vi "Variant Array Decimate.vi"(8 "error in (no error)":errorcluster, 11 "N Dim Array":variant) -> (0 "error out":errorcluster, 1 "Variant Array Type":variant, 2 "Element Type":variant, 3 "Array of Variant Arrays":variant[](array[variant]))   [LabVIEW 2018, in "labview_json.lvlib"]
uses:
  labview_json.lvlib
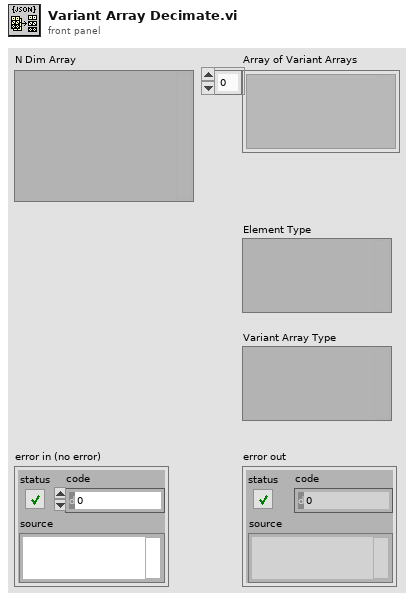
[diagram p1: front panel]
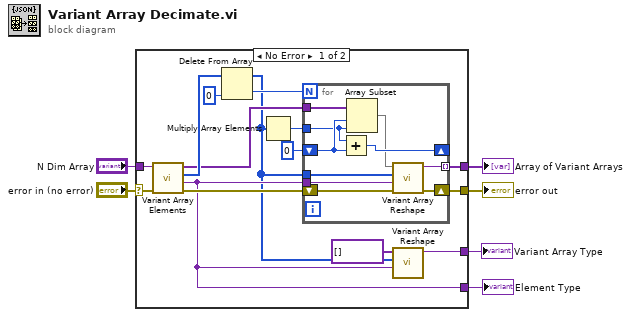
[diagram p0: block diagram]
diagram:
  n1 = case shown="No Error" "error in (no error)" {
    selector: "error in (no error)" -> [w20 w32]
    tunnel: "N Dim Array" -> [w21 _]
    tunnel: [w14 w32] -> w4
    tunnel: [w13 _] -> w3
    tunnel: [w10 _] -> w2
    tunnel: [w7 _] -> w1
    frame No Error {
      n2 = call "Variant Array Elements.vi"("error in (no error)"=w20, "N Dim Array"=w21) -> ("error out"=w12:errorcluster, "Element Type"=w10:variant, "Sizes"=w19:i32[], "Elements"=w11:variant[])  [unwired: 6 in]
      n3 = Delete From Array(array=w19, index=0) -> (deleted portion=w15:i32, array with subset deleted=w9:i32[])  [unwired: 1 in]
      n4 = Multiply Array Elements(1:w9) -> (0:w16:i32)
      n5 = for {
        N: w15 -> [_]
        tunnel: w11 -> [w31]
        shift-right: [w28] -> _
        shift-left: 0 -> [w30]
        tunnel: w16 -> [w29]
        tunnel: w9 -> [w25]
        shift-right: [w26] -> w14
        shift-left: w12 -> [w27]
        tunnel: [w24] -> w13 mode=indexing
        tunnel: w10 -> [w22]
        n6 = Add(x=w29, y=w30) -> (x+y=w28:i32)
        n7 = Array Subset(array=w31, index=w30, length=w29) -> (w23:variant[])
        n8 = call "Variant Array Reshape.vi"("error in (no error)"=w27, "Default Element Type"=w22, "Sizes"=w25, "Elements"=w23) -> ("error out"=w26:errorcluster, "N Dim Array"=w24:variant)  [unwired: 6 in]
      }
      n9 = call "Variant Array Reshape.vi"("Default Element Type"=w10, "Sizes"=w9, "Elements"=variant[] []) -> ("N Dim Array"=w7:variant)  [unwired: 7 in, 1 out]
    }
    frame Error {
    }
  }
  "Array of Variant Arrays" <- w3
  "error out" <- w4
  "Element Type" <- w2
  "Variant Array Type" <- w1
